vi "시험.vi"() -> ()   [LabVIEW 2012]
panel:
  out "합계":i32
  out "부분이 삭제된 배열":i32[][](array[numeric])
  out "배열 2":i32[][](array[numeric])
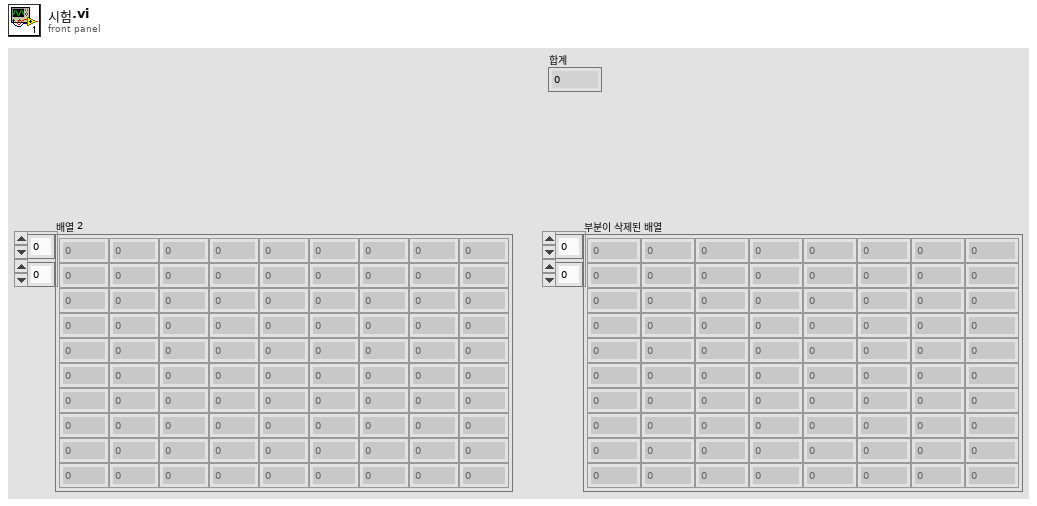
[diagram p1: front panel]
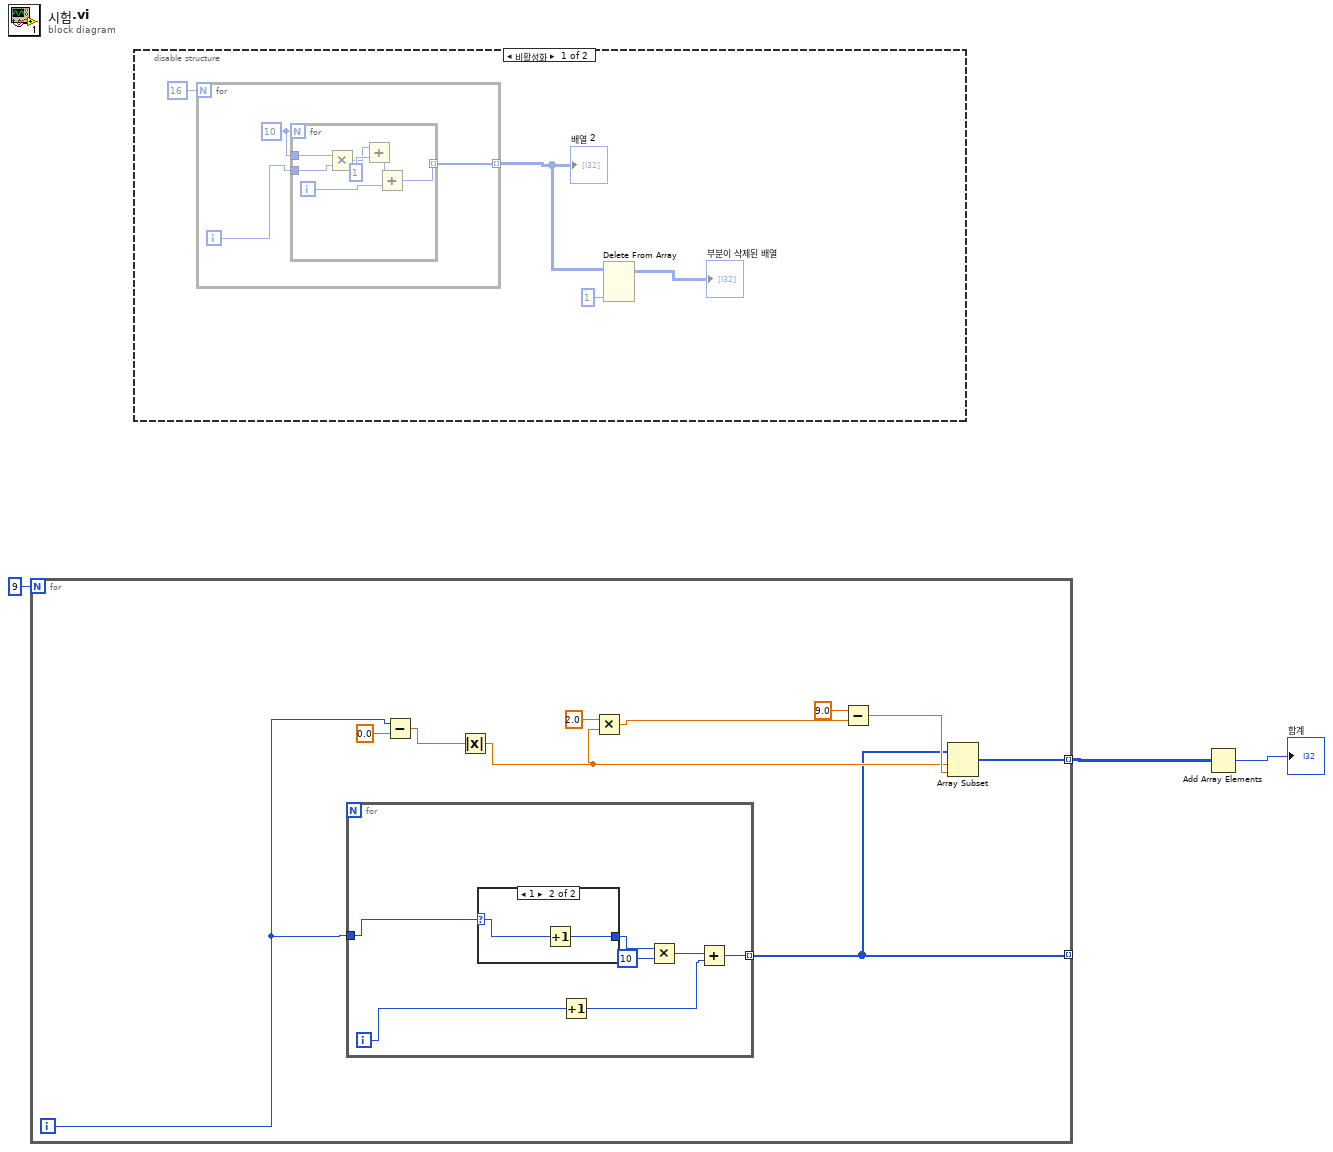
[diagram p0: block diagram]
diagram:
  n1 = for {
    N: 9 -> [_]
    tunnel: [w5] -> _ mode=indexing
    tunnel: [w4] -> w2 mode=indexing
    i -> [w12]
    n2 = for {
      tunnel: w12 -> [w20]
      tunnel: [w14] -> w5 mode=indexing
      i -> [w15]
      n3 = case shown="1" w20 {
        selector: w20 -> [_ w22]
        tunnel: [_ w21] -> w19
        frame 0, Default {
        }
        frame 1 {
          n4 = Increment(x=w22) -> (x+1=w21:i32)
        }
      }
      n5 = Increment(x=w15) -> (x+1=w16:i32)
      n6 = Multiply(x=w19, y=10) -> (x*y=w17:i32)
      n7 = Add(x=w17, y=w16) -> (x+y=w14:i32)
    }
    n8 = Subtract(x=w12, y=0.0) -> (x-y=w11:dbl)
    n9 = Absolute Value(x=w11) -> (abs(x)=w6:dbl)
    n10 = Multiply(x=2.0, y=w6) -> (x*y=w9:dbl)
    n11 = Subtract(x=9.0, y=w9) -> (x-y=w7:dbl)
    n12 = Array Subset(array=w5, index=w6, length=w7) -> (w4:i32[])
  }
  n13 = disable-structure shown="비활성화" {
    frame Disabled {
      n14 = for {
        N: 16 -> [_]
        tunnel: [w29] -> w25 mode=indexing
        i -> [w28]
        w27 = 10
        n15 = for {
          N: w27 -> [_]
          tunnel: [w36] -> w29 mode=indexing
          tunnel: w28 -> [w34]
          tunnel: w27 -> [w32]
          i -> [w35]
          n16 = Multiply(x=w32, y=w34) -> (x*y=w30:i32)
          n17 = Add(x=w30, y=1) -> (x+y=w33:i32)
          n18 = Add(x=w33, y=w35) -> (x+y=w36:i32)
        }
      }
      "배열 2" <- w25
      n19 = Delete From Array(array=w25, index (col)=1 ("비활성화된 인덱스 (열)")) -> (array with subset deleted=→"부분이 삭제된 배열":i32[][])  [unwired: 2 in, 1 out]
    }
    frame Enabled {
    }
  }
  n20 = Add Array Elements(numeric array=w2) -> (sum=→"합계":i32)
